vi "Autonomous Independent.vi"() -> ()   [LabVIEW 2014]
doc: "This VI is called when autonomous begins, and will automatically be terminated when autonomous ends. You can carry out timed or sensor driven robot movement independently without needing to return to the caller."
uses:
  <vilib>/Rock Robotics/WPI/Joystick/WPI_JoystickGetSetRefNum.vi
  <vilib>/Rock Robotics/WPI/RobotDrive/WPI_RobotDriveGetSetRefNum.vi
  Robot Global Data.vi
  <vilib>/Rock Robotics/WPI/RobotDrive/WPI_RobotDriveArcadeDrive_Standard(NoSaturation).vi
  <vilib>/Rock Robotics/Network Tables/SD Write Boolean.vi
panel:
  out "Auto 6":bool=TRUE
  out "Auto 5":bool=TRUE
  in  "Array of robot movements 6":T1(array[cluster])=[{"X Joystick Value"=0.7, "Y Joystick Value"=0.0, "Delay (sec)"=2.0, "Movement Name"="90 turn", "Joystick Button 1"=FALSE, "Joystick Button 2"=FALSE, "Joystick Button 3"=FALSE, "Joystick Button 4"=FALSE, "Joystick Button 5"=FALSE, "Joystick Button 6"=FALSE, "Joystick Button 7"=FALSE, "Joystick Button 8"=FALSE, "Joystick Button 9"=FALSE, "Joystick Button 10"=FALSE, "Joystick Button 11"=FALSE, "Joystick Button 12"=FALSE}, {"X Joystick Value"=0.0, "Y Joystick Value"=0.0, "Delay (sec)"=0.0, "Movement Name"="Stop", "Joystick Button 1"=FALSE, "Joystick Button 2"=FALSE, "Joystick Button 3"=FALSE, "Joystick Button 4"=FALSE, "Joystick Button 5"=FALSE, "Joystick Button 6"=FALSE, "Joystick Button 7"=FALSE, "Joystick Button 8"=FALSE, "Joystick Button 9"=FALSE, "Joystick Button 10"=FALSE, "Joystick Button 11"=FALSE, "Joystick Button 12"=FALSE}] {"Y Joystick Value" scale=1.0..-1.0; "X Joystick Value" scale=-1.0..1.0}
  in  "Array of robot movements 5":T1(array[cluster])=[{"X Joystick Value"=0.17, "Y Joystick Value"=-0.45, "Delay (sec)"=1.2, "Movement Name"="Drive 600mm", "Joystick Button 1"=FALSE, "Joystick Button 2"=FALSE, "Joystick Button 3"=FALSE, "Joystick Button 4"=FALSE, "Joystick Button 5"=FALSE, "Joystick Button 6"=FALSE, "Joystick Button 7"=FALSE, "Joystick Button 8"=FALSE, "Joystick Button 9"=FALSE, "Joystick Button 10"=FALSE, "Joystick Button 11"=FALSE, "Joystick Button 12"=FALSE}, {"X Joystick Value"=0.0, "Y Joystick Value"=0.0, "Delay (sec)"=0.0, "Movement Name"="Stop", "Joystick Button 1"=FALSE, "Joystick Button 2"=FALSE, "Joystick Button 3"=FALSE, "Joystick Button 4"=FALSE, "Joystick Button 5"=FALSE, "Joystick Button 6"=FALSE, "Joystick Button 7"=FALSE, "Joystick Button 8"=FALSE, "Joystick Button 9"=FALSE, "Joystick Button 10"=FALSE, "Joystick Button 11"=FALSE, "Joystick Button 12"=FALSE}] {"Y Joystick Value" scale=1.0..-1.0; "X Joystick Value" scale=-1.0..1.0}
  out "Auto 4":bool=TRUE
  out "Auto 3":bool=TRUE
  out "Auto 2":bool=TRUE
  out "Auto 1":bool=TRUE
  in  "Array of robot movements 4":T1(array[cluster])=[{"X Joystick Value"=0.33, "Y Joystick Value"=-0.75, "Delay (sec)"=5.0, "Movement Name"="Drive to Auto", "Joystick Button 1"=FALSE, "Joystick Button 2"=FALSE, "Joystick Button 3"=FALSE, "Joystick Button 4"=FALSE, "Joystick Button 5"=FALSE, "Joystick Button 6"=FALSE, "Joystick Button 7"=FALSE, "Joystick Button 8"=FALSE, "Joystick Button 9"=FALSE, "Joystick Button 10"=FALSE, "Joystick Button 11"=FALSE, "Joystick Button 12"=FALSE}, {"X Joystick Value"=0.0, "Y Joystick Value"=0.0, "Delay (sec)"=0.0, "Movement Name"="Stop", "Joystick Button 1"=FALSE, "Joystick Button 2"=FALSE, "Joystick Button 3"=FALSE, "Joystick Button 4"=FALSE, "Joystick Button 5"=FALSE, "Joystick Button 6"=FALSE, "Joystick Button 7"=FALSE, "Joystick Button 8"=FALSE, "Joystick Button 9"=FALSE, "Joystick Button 10"=FALSE, "Joystick Button 11"=FALSE, "Joystick Button 12"=FALSE}] {"Y Joystick Value" scale=1.0..-1.0; "X Joystick Value" scale=-1.0..1.0}
  in  "Array of robot movements 3":T1(array[cluster])=[{"X Joystick Value"=0.7, "Y Joystick Value"=0.0, "Delay (sec)"=1.4, "Movement Name"="Turn 90' right", "Joystick Button 1"=FALSE, "Joystick Button 2"=FALSE, "Joystick Button 3"=FALSE, "Joystick Button 4"=FALSE, "Joystick Button 5"=FALSE, "Joystick Button 6"=FALSE, "Joystick Button 7"=FALSE, "Joystick Button 8"=FALSE, "Joystick Button 9"=FALSE, "Joystick Button 10"=FALSE, "Joystick Button 11"=FALSE, "Joystick Button 12"=FALSE}, {"X Joystick Value"=0.33, "Y Joystick Value"=-0.75, "Delay (sec)"=3.0, "Movement Name"="Drive to Auto", "Joystick Button 1"=FALSE, "Joystick Button 2"=FALSE, "Joystick Button 3"=FALSE, "Joystick Button 4"=FALSE, "Joystick Button 5"=FALSE, "Joystick Button 6"=FALSE, "Joystick Button 7"=FALSE, "Joystick Button 8"=FALSE, "Joystick Button 9"=FALSE, "Joystick Button 10"=FALSE, "Joystick Button 11"=FALSE, "Joystick Button 12"=FALSE}, {"X Joystick Value"=0.0, "Y Joystick Value"=0.0, "Delay (sec)"=0.0, "Movement Name"="Stop", "Joystick Button 1"=FALSE, "Joystick Button 2"=FALSE, "Joystick Button 3"=FALSE, "Joystick Button 4"=FALSE, "Joystick Button 5"=FALSE, "Joystick Button 6"=FALSE, "Joystick Button 7"=FALSE, "Joystick Button 8"=FALSE, "Joystick Button 9"=FALSE, "Joystick Button 10"=FALSE, "Joystick Button 11"=FALSE, "Joystick Button 12"=FALSE}] {"Y Joystick Value" scale=1.0..-1.0; "X Joystick Value" scale=-1.0..1.0}
  in  "Array of robot movements 2":T1(array[cluster])=[{"X Joystick Value"=0.0, "Y Joystick Value"=0.0, "Delay (sec)"=0.5, "Movement Name"="Lift arm 4 bin", "Joystick Button 1"=FALSE, "Joystick Button 2"=FALSE, "Joystick Button 3"=FALSE, "Joystick Button 4"=FALSE, "Joystick Button 5"=FALSE, "Joystick Button 6"=FALSE, "Joystick Button 7"=FALSE, "Joystick Button 8"=TRUE, "Joystick Button 9"=FALSE, "Joystick Button 10"=FALSE, "Joystick Button 11"=FALSE, "Joystick Button 12"=FALSE}, {"X Joystick Value"=0.0, "Y Joystick Value"=0.0, "Delay (sec)"=4.55, "Movement Name"="Wait for arm", "Joystick Button 1"=FALSE, "Joystick Button 2"=FALSE, "Joystick Button 3"=FALSE, "Joystick Button 4"=FALSE, "Joystick Button 5"=FALSE, "Joystick Button 6"=FALSE, "Joystick Button 7"=FALSE, "Joystick Button 8"=FALSE, "Joystick Button 9"=FALSE, "Joystick Button 10"=FALSE, "Joystick Button 11"=FALSE, "Joystick Button 12"=FALSE}, {"X Joystick Value"=0.33, "Y Joystick Value"=-0.75, "Delay (sec)"=5.0, "Movement Name"="Drive to Auto", "Joystick Button 1"=FALSE, "Joystick Button 2"=FALSE, "Joystick Button 3"=FALSE, "Joystick Button 4"=FALSE, "Joystick Button 5"=FALSE, "Joystick Button 6"=FALSE, "Joystick Button 7"=FALSE, "Joystick Button 8"=FALSE, "Joystick Button 9"=FALSE, "Joystick Button 10"=FALSE, "Joystick Button 11"=FALSE, "Joystick Button 12"=FALSE}, {"X Joystick Value"=0.0, "Y Joystick Value"=0.0, "Delay (sec)"=0.0, "Movement Name"="Stop", "Joystick Button 1"=FALSE, "Joystick Button 2"=FALSE, "Joystick Button 3"=FALSE, "Joystick Button 4"=FALSE, "Joystick Button 5"=FALSE, "Joystick Button 6"=FALSE, "Joystick Button 7"=FALSE, "Joystick Button 8"=FALSE, "Joystick Button 9"=FALSE, "Joystick Button 10"=FALSE, "Joystick Button 11"=FALSE, "Joystick Button 12"=FALSE}] {"Y Joystick Value" scale=1.0..-1.0; "X Joystick Value" scale=-1.0..1.0}
  in  "Array of robot movements 1":T1(array[cluster])=[{"X Joystick Value"=0.0, "Y Joystick Value"=0.0, "Delay (sec)"=0.5, "Movement Name"="lift arm 4 bin", "Joystick Button 1"=FALSE, "Joystick Button 2"=FALSE, "Joystick Button 3"=FALSE, "Joystick Button 4"=FALSE, "Joystick Button 5"=FALSE, "Joystick Button 6"=FALSE, "Joystick Button 7"=FALSE, "Joystick Button 8"=TRUE, "Joystick Button 9"=FALSE, "Joystick Button 10"=FALSE, "Joystick Button 11"=FALSE, "Joystick Button 12"=FALSE}, {"X Joystick Value"=0.0, "Y Joystick Value"=0.0, "Delay (sec)"=4.55, "Movement Name"="Wait for arm", "Joystick Button 1"=FALSE, "Joystick Button 2"=FALSE, "Joystick Button 3"=FALSE, "Joystick Button 4"=FALSE, "Joystick Button 5"=FALSE, "Joystick Button 6"=FALSE, "Joystick Button 7"=FALSE, "Joystick Button 8"=FALSE, "Joystick Button 9"=FALSE, "Joystick Button 10"=FALSE, "Joystick Button 11"=FALSE, "Joystick Button 12"=FALSE}, {"X Joystick Value"=0.7, "Y Joystick Value"=0.0, "Delay (sec)"=1.4, "Movement Name"="Turn 90 right", "Joystick Button 1"=FALSE, "Joystick Button 2"=FALSE, "Joystick Button 3"=FALSE, "Joystick Button 4"=FALSE, "Joystick Button 5"=FALSE, "Joystick Button 6"=FALSE, "Joystick Button 7"=FALSE, "Joystick Button 8"=FALSE, "Joystick Button 9"=FALSE, "Joystick Button 10"=FALSE, "Joystick Button 11"=FALSE, "Joystick Button 12"=FALSE}, {"X Joystick Value"=0.33, "Y Joystick Value"=-0.75, "Delay (sec)"=3.0, "Movement Name"="Drive to Auto", "Joystick Button 1"=FALSE, "Joystick Button 2"=FALSE, "Joystick Button 3"=FALSE, "Joystick Button 4"=FALSE, "Joystick Button 5"=FALSE, "Joystick Button 6"=FALSE, "Joystick Button 7"=FALSE, "Joystick Button 8"=FALSE, "Joystick Button 9"=FALSE, "Joystick Button 10"=FALSE, "Joystick Button 11"=FALSE, "Joystick Button 12"=FALSE}, {"X Joystick Value"=0.0, "Y Joystick Value"=0.0, "Delay (sec)"=0.0, "Movement Name"="Stop", "Joystick Button 1"=FALSE, "Joystick Button 2"=FALSE, "Joystick Button 3"=FALSE, "Joystick Button 4"=FALSE, "Joystick Button 5"=FALSE, "Joystick Button 6"=FALSE, "Joystick Button 7"=FALSE, "Joystick Button 8"=FALSE, "Joystick Button 9"=FALSE, "Joystick Button 10"=FALSE, "Joystick Button 11"=FALSE, "Joystick Button 12"=FALSE}] {"Y Joystick Value" scale=1.0..-1.0; "X Joystick Value" scale=-1.0..1.0}
  # "######################################################\n    #                                                      #\n    #   SAFETY NOTICE: MAKE SURE THAT EACH ARRAY ON THIS   #\n    #   FRONT PANEL IS DISPLAYING A \"GREYED OUT\" (DEFAULT) #\n    #   ELEMENT ON THE RIGHT                               #\n    #                                                      #\n     ######################################################\n\nNOTE#1: any changes made here are not permanent until you have selected the modified array, right-click and select \"Data Operations\" > \"Make Current Value Default\"\n\nNOTE#2: to add an extra \"element\" to one of the arrays simply select the array and drag the right side further to the right, a new element will be added to the end of the array. Alternatively, select an existing element then right click and select \"Data Operations\" > \"Insert Element Before\".\n\nNOTE#3: to remove an element you must explicitly delete the element, DO NOT be tempted to just grab the end of the array and drag it to the left as all that does is limit what is visible on screen. To delete an element select it then right-click and select \"Data Operations\" > \"Delete Element\"."
  # "AUTO 1:\n1 bin\n1 tote"
  # "Start around left bin\nwith arm down"
  # "AUTO 2:\n1 bin\n2 totes"
  # "starts around middle bin\nwith arm down"
  # "AUTO 3:\nReady 1 tote"
  # "Starts around left tote\nwith arm down"
  # "Be sure to right-click and choose Data Operations>>Make Current Value default if you want to save the array values with the VI"
  # "AUTO 4:\nAuto Zone"
  # "Start backed up to left tote\nArm doesn't matter"
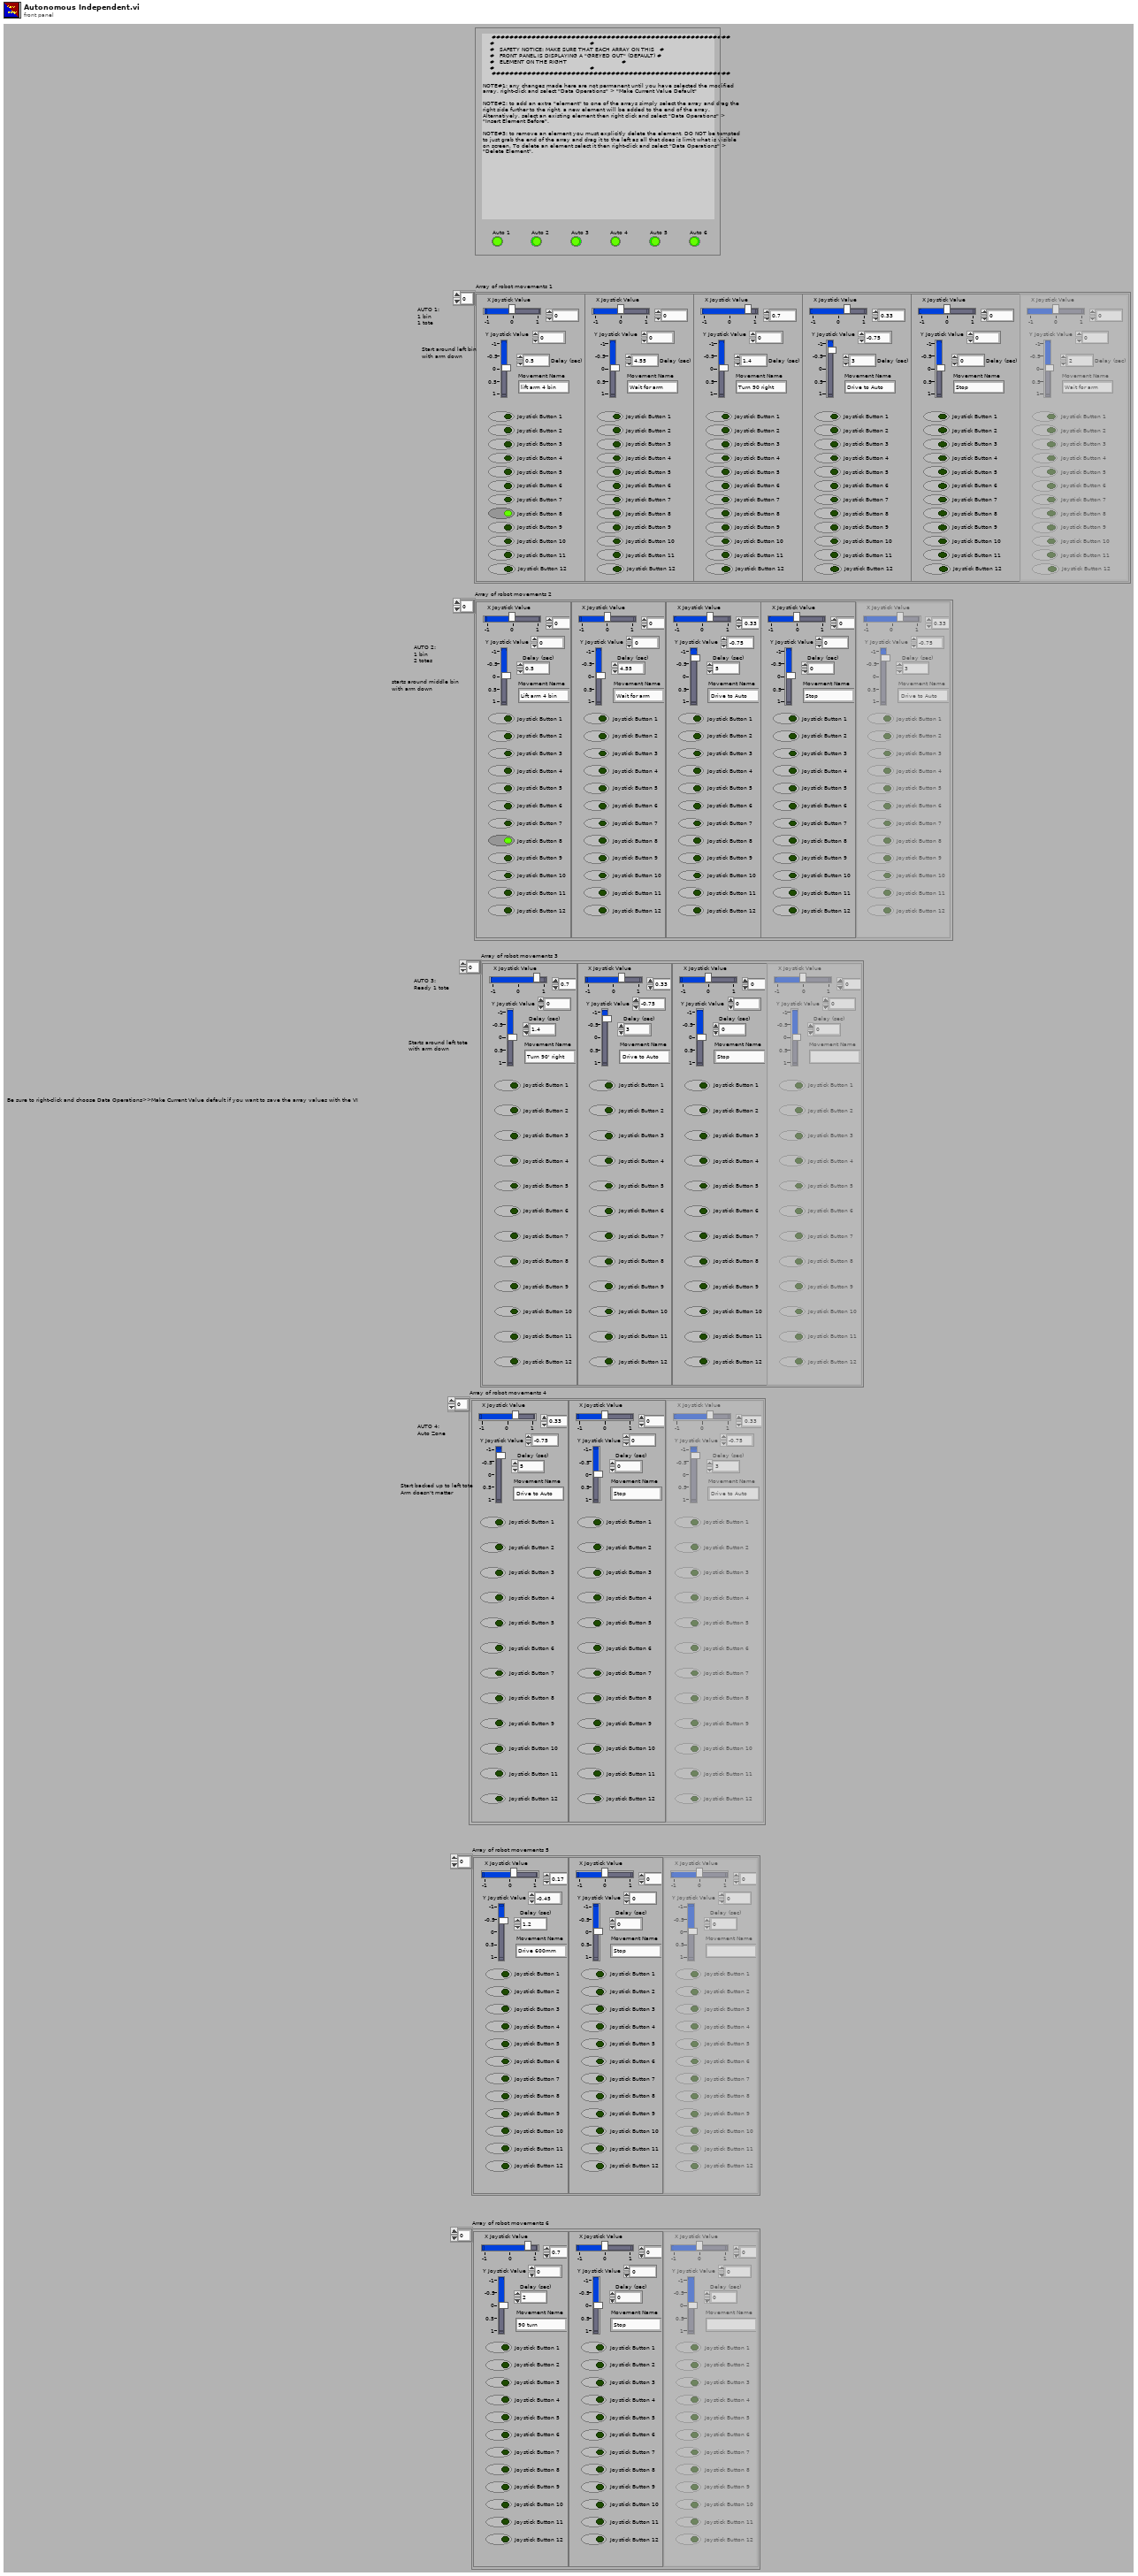
[diagram p1: front panel]
types:
  T1 = cluster{"X Joystick Value":dbl, "Y Joystick Value":dbl, "Delay (sec)":dbl, "Movement Name":string, "Joystick Button 1":bool, "Joystick Button 2":bool, "Joystick Button 3":bool, "Joystick Button 4":bool, "Joystick Button 5":bool, "Joystick Button 6":bool, "Joystick Button 7":bool, "Joystick Button 8":bool, "Joystick Button 9":bool, "Joystick Button 10":bool, "Joystick Button 11":bool, "Joystick Button 12":bool}[]
  T2 = typedef "WPI_JoystickDevRef.ctl" = cluster{"Device":T3}
  T3 = typedef "WPI_JoystickDeviceEnum.ctl" = enum16{"USB 0", "USB 1", "USB 2", "USB 3", "USB 4", "USB 5"}
  T4 = typedef "WPI_DigitalInputDevRef.ctl" = cluster{"DevStatus":errorcluster, "DIO Channel":T5, "Controller":T6}
  T5 = typedef "FPGA_DIOChannel.ctl" = enum8{"DIO 0", "DIO 1", "DIO 2", "DIO 3", "DIO 4", "DIO 5", "DIO 6", "DIO 7", "DIO 8", "DIO 9", "DIO MXP 0", "DIO MXP 1", "DIO MXP 2", "DIO MXP 3", "DIO MXP 4", "DIO MXP 5", "DIO MXP 6", "DIO MXP 7", "DIO MXP 8", "DIO MXP 9", "DIO MXP 10", "DIO MXP 11", "DIO MXP 12", "DIO MXP 13", "DIO MXP 14", "DIO MXP 15", "Invalid"}
  T6 = typedef "FPGA_TypedefDigitalModule.ctl" = enum16{"Controller 1"}
  T7 = typedef "WPI_RobotDriveDevRef.ctl" = cluster{"DevStatus":errorcluster, "Motors[]":T8[], "Square Inputs":bool, "Max Output":dbl}
  T8 = typedef "WPI_MotorControlDeviceRef.ctl" = cluster{"DeviceStatus":errorcluster, "Type":T9, "PWM":cluster{"Controller":T6, "PWM Channel":T10, "DeadBand":T11}, "CAN":cluster{"Device Number":u8, "Control Mode":T12, "Semaphore":T13, "Max Vout":dbl, "TalonSRX Control Mode":T14}, "Invert":bool, "TransformRef":T15, "InvTransformRef":T15}
  T9 = typedef "WPI_MotorControlType.ctl" = enum16{"PWM", "CAN", "CANTalonSRX"}
  T10 = typedef "FPGA_DIOPWMChannel.ctl" = enum8{"PWM 0", "PWM 1", "PWM 2", "PWM 3", "PWM 4", "PWM 5", "PWM 6", "PWM 7", "PWM 8", "PWM 9", "PWM MXP 0", "PWM MXP 1", "PWM MXP 2", "PWM MXP 3", "PWM MXP 4", "PWM MXP 5", "PWM MXP 6", "PWM MXP 7", "PWM MXP 8", "PWM MXP 9", "Invalid"}
  T11 = typedef "WPI_PWMDeadband.ctl" = cluster{"Name":string, "maxPositivePwm":i32, "minPositivePwm":i32, "centerPwm":i32, "maxNegativePwm":i32, "minNegativePwm":i32, "angularRange":u16}
  T12 = typedef "WPI_CANJaguar_ControlMode.ctl" = enum8{"Percent VBus", "Current", "Speed", "Position", "Voltage"}
  T13 = typedef "Semaphore RefNum" = refnum<k1>
  T14 = typedef "WPI_CANTalonSRX_APIControlMode.ctl" = enum8{"Percent VBus", "Speed", "Position", "Slave", "Unchanged / Invalid"}
  T15 = typedef "WPI_PWMTransform_ConPane.ctl" = refnum<vi>
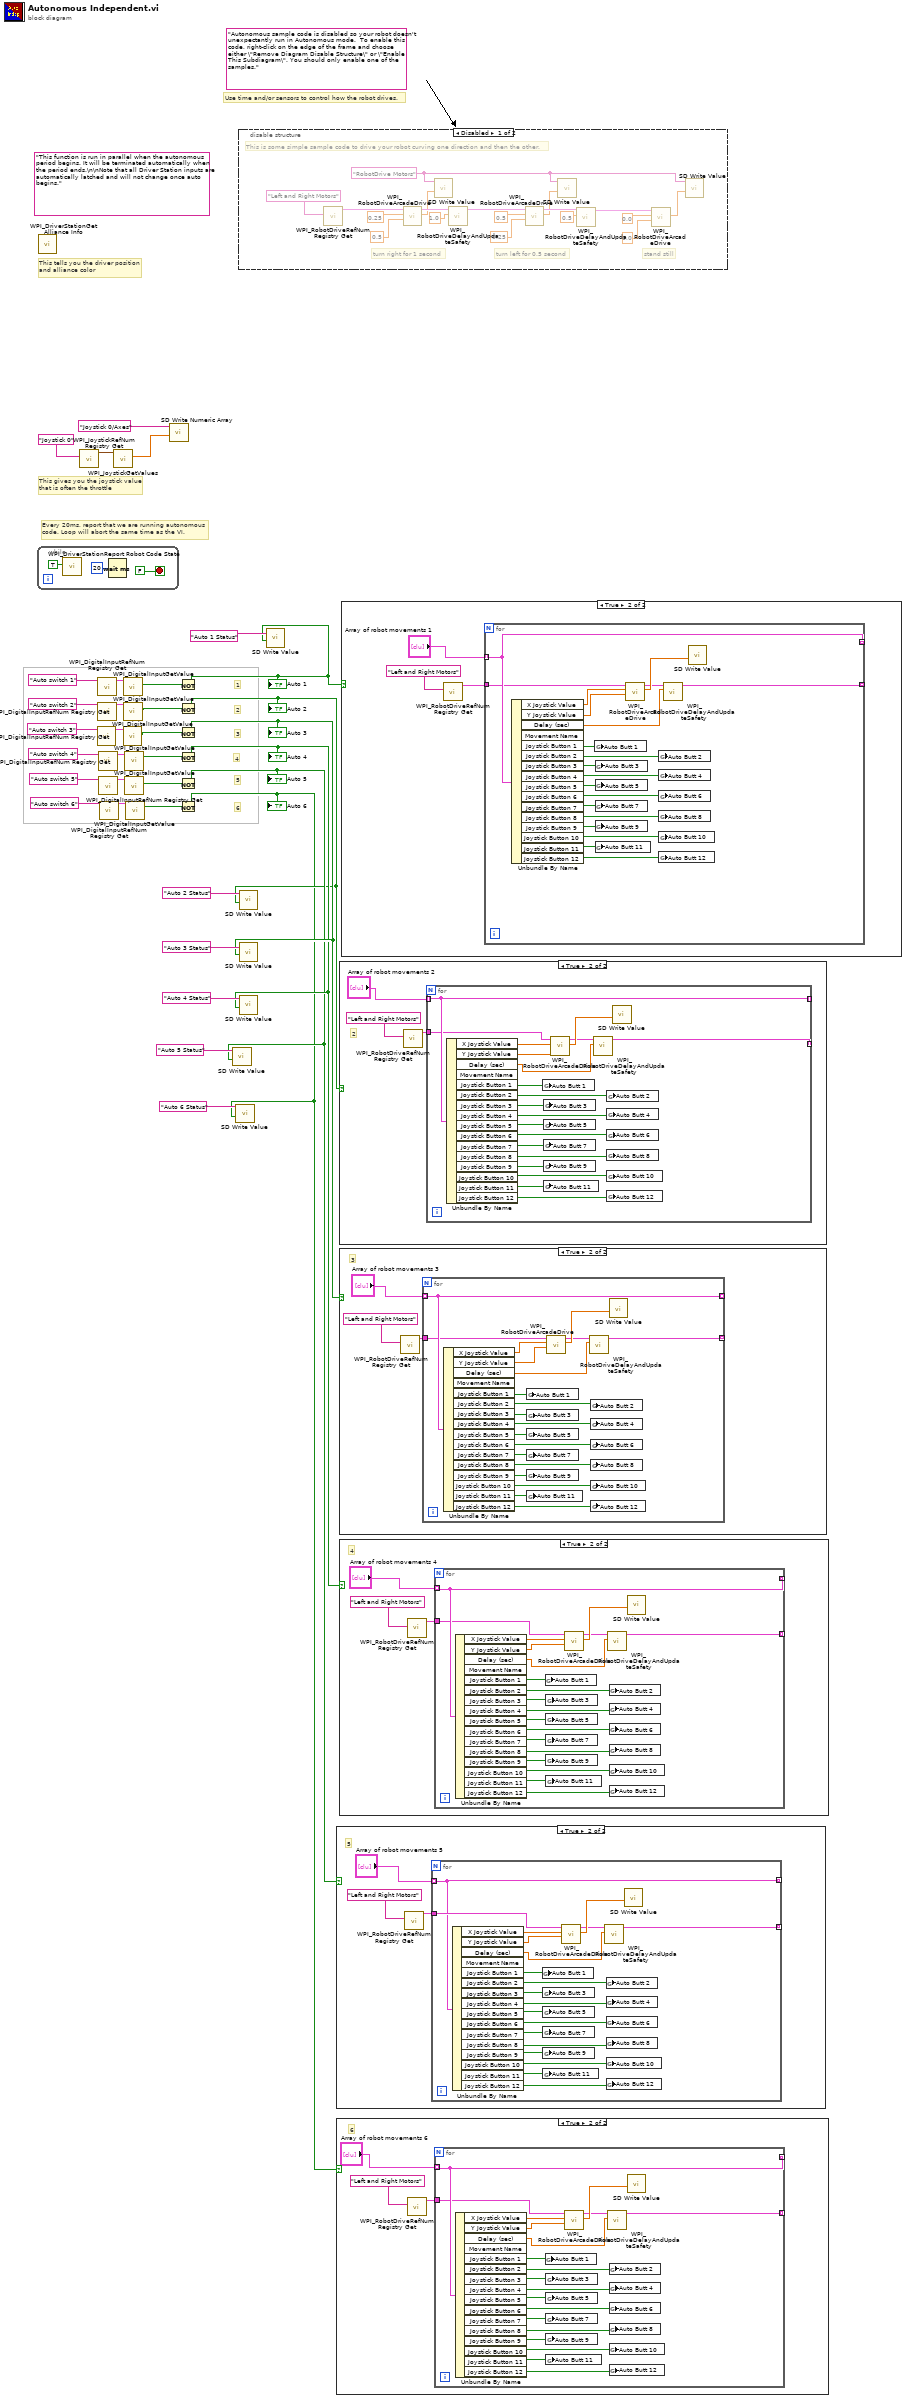
[diagram p0: block diagram]
diagram:
  (unwired) "Autonomous sample code is disabled so your robot doesn't unexpectantly run in Autonomous mode.  To enable this code, right-click on the edge of the frame and choose either \"Remove Diagram Disable Structure\" or \"Enable This Subdiagram\". You should only enable one of the samples."
  (unwired) "This function is run in parallel when the autonomous period begins. It will be terminated automatically when the period ends.\n\nNote that all Driver Station inputs are automatically latched and will not change once auto begins."
  # "6"
  # "5"
  # "4"
  # "3"
  # "2"
  # "1"
  # "Every 20ms, report that we are running autonomous\ncode. Loop will abort the same time as the VI."
  # "This gives you the joystick value\nthat is often the throttle"
  # "Use time and/or sensors to control how the robot drives."
  # "This tells you the driver position\nand alliance color"
  n1 = while {
    stop <- FALSE stop-if-true
    n2 = call <vilib>:"WPI_DriverStationReport Robot Code State.vi"("Autonomous"=TRUE) -> ()  [unwired: 10 in, 1 out]
    n3 = Wait (ms)(milliseconds to wait=u32 20) -> ()  [unwired: 1 out]
  }
  n4 = call <vilib>:"WPI_DriverStationGet Alliance Info.vi"() -> ()  [unwired: 12 out]
  n5 = call <vilib>:"WPI_JoystickRefNum Registry Get.vi"("refnum name"="Joystick 0") -> ("JoystickDevRef"=w33:T2)  [unwired: 1 in, 9 out]
  n6 = call <vilib>:"WPI_DigitalInputRefNum Registry Get.vi"("refnum name"="Auto switch 3") -> ("DigitalInputDevRef"=w15:T4)  [unwired: 9 in, 1 out]
  n7 = call <vilib>:"WPI_DigitalInputRefNum Registry Get.vi"("refnum name"="Auto switch 1") -> ("DigitalInputDevRef"=w27:T4)  [unwired: 9 in, 1 out]
  n8 = call <vilib>:"WPI_DigitalInputRefNum Registry Get.vi"("refnum name"="Auto switch 2") -> ("DigitalInputDevRef"=w28:T4)  [unwired: 9 in, 1 out]
  n9 = call <vilib>:"WPI_DigitalInputRefNum Registry Get.vi"("refnum name"="Auto switch 4") -> ("DigitalInputDevRef"=w16:T4)  [unwired: 9 in, 1 out]
  n10 = call <vilib>:"WPI_DigitalInputRefNum Registry Get.vi"("refnum name"="Auto switch 5") -> ("DigitalInputDevRef"=w14:T4)  [unwired: 9 in, 1 out]
  n11 = call <vilib>:"WPI_DigitalInputRefNum Registry Get.vi"("refnum name"="Auto switch 6") -> ("DigitalInputDevRef"=w13:T4)  [unwired: 9 in, 1 out]
  n12 = call <vilib>:"WPI_JoystickGetValues.vi"("JoystickDevRef"=w33) -> ("Axes"=w31:dbl[])  [unwired: 6 in, 4 out]
  n13 = call <vilib>:"WPI_DigitalInputGetValue.vi"("DigitalInputDevRef"=w15) -> ("Value"=w10:bool)  [unwired: 8 in, 2 out]
  n14 = call <vilib>:"WPI_DigitalInputGetValue.vi"("DigitalInputDevRef"=w27) -> ("Value"=w12:bool)  [unwired: 8 in, 2 out]
  n15 = call <vilib>:"WPI_DigitalInputGetValue.vi"("DigitalInputDevRef"=w28) -> ("Value"=w11:bool)  [unwired: 8 in, 2 out]
  n16 = call <vilib>:"WPI_DigitalInputGetValue.vi"("DigitalInputDevRef"=w16) -> ("Value"=w8:bool)  [unwired: 8 in, 2 out]
  n17 = call <vilib>:"WPI_DigitalInputGetValue.vi"("DigitalInputDevRef"=w14) -> ("Value"=w6:bool)  [unwired: 8 in, 2 out]
  n18 = call <vilib>:"WPI_DigitalInputGetValue.vi"("DigitalInputDevRef"=w13) -> ("Value"=w4:bool)  [unwired: 8 in, 2 out]
  n19 = call <vilib>:"SD Write Numeric Array.vi"("Numeric Array"=w31, "Name"="Joystick 0/Axes") -> ()  [unwired: 8 in, 2 out]
  n20 = Not(x=w12) -> (.not. x?=w3:bool)
  "Auto 1" <- w3
  n21 = Not(x=w11) -> (.not. x?=w2:bool)
  "Auto 2" <- w2
  n22 = Not(x=w10) -> (.not. x?=w9:bool)
  "Auto 3" <- w9
  n23 = Not(x=w8) -> (.not. x?=w7:bool)
  "Auto 4" <- w7
  n24 = Not(x=w6) -> (.not. x?=w5:bool)
  "Auto 5" <- w5
  n25 = Not(x=w4) -> (.not. x?=w1:bool)
  "Auto 6" <- w1
  n26 = call-poly <vilib>:"SD Write Value.vi"("Boolean"=w5, "Name"="Auto 5 Status") -> ()  [unwired: 8 in, 2 out]
  n27 = call-poly <vilib>:"SD Write Value.vi"("Boolean"=w1, "Name"="Auto 6 Status") -> ()  [unwired: 8 in, 2 out]
  n28 = disable-structure shown="Disabled" {
    frame Disabled {
      w41 = "RobotDrive Motors" ("Name")
      # "This is some simple sample code to drive your robot curving one direction and then the other."
      # "stand still"
      # "turn left for 0.5 second"
      # "turn right for 1 second"
      n29 = call <vilib>:"WPI_RobotDriveRefNum Registry Get.vi"("refnum name"="Left and Right Motors") -> ("RobotDriveDevRef"=w42:T7)  [unwired: 1 in, 9 out]
      n30 = call-poly <vilib>:"WPI_RobotDriveArcadeDrive.vi"("Y axis value"=0.5 ("X axis value"), "X axis value"=0.25, "RobotDriveDevRef"=w42) -> ("Motor Values"=w40:dbl[], "RobotDriveDevRef"=w49:T7)  [unwired: 1 in, 6 out]
      n31 = call-poly <vilib>:"SD Write Value.vi"("Numeric Array"=w40, "Name"=w41) -> ()  [unwired: 8 in, 2 out]
      n32 = call <vilib>:"WPI_RobotDriveDelayAndUpdateSafety.vi"("Delay (s)"=1.0, "RobotDriveDevRef"=w49) -> ("RobotDriveDevRef 2"=w48:T7)  [unwired: 8 in, 1 out]
      n33 = call-poly <vilib>:"WPI_RobotDriveArcadeDrive.vi"("Y axis value"=0.25 ("X axis value"), "X axis value"=0.5, "RobotDriveDevRef"=w48) -> ("Motor Values"=w39:dbl[], "RobotDriveDevRef"=w47:T7)  [unwired: 1 in, 6 out]
      n34 = call-poly <vilib>:"SD Write Value.vi"("Numeric Array"=w39, "Name"=w41) -> ()  [unwired: 8 in, 2 out]
      n35 = call <vilib>:"WPI_RobotDriveDelayAndUpdateSafety.vi"("Delay (s)"=0.5, "RobotDriveDevRef"=w47) -> ("RobotDriveDevRef 2"=w46:T7)  [unwired: 8 in, 1 out]
      n36 = call-poly <vilib>:"WPI_RobotDriveArcadeDrive.vi"("Y axis value"=0.0 ("X axis value"), "X axis value"=0.0, "RobotDriveDevRef"=w46) -> ("Motor Values"=w38:dbl[])  [unwired: 1 in, 7 out]
      n37 = call-poly <vilib>:"SD Write Value.vi"("Numeric Array"=w38, "Name"=w41) -> ()  [unwired: 8 in, 2 out]
    }
    frame Enabled {
    }
  }
  n38 = call-poly <vilib>:"SD Write Value.vi"("Boolean"=w2, "Name"="Auto 2 Status") -> ()  [unwired: 8 in, 2 out]
  n39 = call-poly <vilib>:"SD Write Value.vi"("Boolean"=w9, "Name"="Auto 3 Status") -> ()  [unwired: 8 in, 2 out]
  n40 = call-poly <vilib>:"SD Write Value.vi"("Boolean"=w7, "Name"="Auto 4 Status") -> ()  [unwired: 8 in, 2 out]
  n41 = call-poly <vilib>:"SD Write Value.vi"("Boolean"=w3, "Name"="Auto 1 Status") -> ()  [unwired: 8 in, 2 out]
  n42 = case shown="True" w5 {
    frame False {
    }
    frame True {
      # "5"
      n43 = call <vilib>:"WPI_RobotDriveRefNum Registry Get.vi"("refnum name"="Left and Right Motors") -> ("RobotDriveDevRef"=w57:T7)  [unwired: 1 in, 9 out]
      n44 = for {
        tunnel: "Array of robot movements 5" -> [w59] mode=indexing
        tunnel: [w59] -> _ mode=indexing
        tunnel: w57 -> [w76]
        tunnel: [w73] -> _ mode=indexing
        n45 = Unbundle By Name(w59) -> ("X Joystick Value"=w75:dbl, "Y Joystick Value"=w74:dbl, "Delay (sec)"=w72:dbl, "Joystick Button 1"=w71:bool, "Joystick Button 2"=w65:bool, "Joystick Button 3"=w70:bool, "Joystick Button 4"=w64:bool, "Joystick Button 5"=w69:bool, "Joystick Button 6"=w63:bool, "Joystick Button 7"=w68:bool, "Joystick Button 8"=w62:bool, "Joystick Button 9"=w67:bool, "Joystick Button 10"=w61:bool, "Joystick Button 11"=w66:bool, "Joystick Button 12"=w60:bool)  [unwired: 1 out]
        n46 = global write "Robot Global Data.vi" "Auto Butt 1"(w71) -> ()
        n47 = global write "Robot Global Data.vi" "Auto Butt 3"(w70) -> ()
        n48 = global write "Robot Global Data.vi" "Auto Butt 5"(w69) -> ()
        n49 = global write "Robot Global Data.vi" "Auto Butt 7"(w68) -> ()
        n50 = global write "Robot Global Data.vi" "Auto Butt 9"(w67) -> ()
        n51 = global write "Robot Global Data.vi" "Auto Butt 11"(w66) -> ()
        n52 = call-poly <vilib>:"WPI_RobotDriveArcadeDrive.vi"("Y axis value"=w74, "X axis value"=w75, "RobotDriveDevRef"=w76) -> ("Motor Values"=w78:dbl[], "RobotDriveDevRef"=w77:T7)  [unwired: 1 in, 6 out]
        n53 = call <vilib>:"WPI_RobotDriveDelayAndUpdateSafety.vi"("Delay (s)"=w72, "RobotDriveDevRef"=w77) -> ("RobotDriveDevRef 2"=w73:T7)  [unwired: 8 in, 1 out]
        n54 = global write "Robot Global Data.vi" "Auto Butt 2"(w65) -> ()
        n55 = global write "Robot Global Data.vi" "Auto Butt 4"(w64) -> ()
        n56 = global write "Robot Global Data.vi" "Auto Butt 6"(w63) -> ()
        n57 = global write "Robot Global Data.vi" "Auto Butt 8"(w62) -> ()
        n58 = global write "Robot Global Data.vi" "Auto Butt 10"(w61) -> ()
        n59 = global write "Robot Global Data.vi" "Auto Butt 12"(w60) -> ()
        n60 = call-poly <vilib>:"SD Write Value.vi"("Numeric Array"=w78) -> ()  [unwired: 9 in, 2 out]
      }
    }
  }
  n61 = case shown="True" w1 {
    frame False {
    }
    frame True {
      # "6"
      n62 = call <vilib>:"WPI_RobotDriveRefNum Registry Get.vi"("refnum name"="Left and Right Motors") -> ("RobotDriveDevRef"=w80:T7)  [unwired: 1 in, 9 out]
      n63 = for {
        tunnel: "Array of robot movements 6" -> [w101] mode=indexing
        tunnel: [w101] -> _ mode=indexing
        tunnel: w80 -> [w98]
        tunnel: [w95] -> _ mode=indexing
        n64 = Unbundle By Name(w101) -> ("X Joystick Value"=w97:dbl, "Y Joystick Value"=w96:dbl, "Delay (sec)"=w94:dbl, "Joystick Button 1"=w93:bool, "Joystick Button 2"=w87:bool, "Joystick Button 3"=w92:bool, "Joystick Button 4"=w86:bool, "Joystick Button 5"=w91:bool, "Joystick Button 6"=w85:bool, "Joystick Button 7"=w90:bool, "Joystick Button 8"=w84:bool, "Joystick Button 9"=w89:bool, "Joystick Button 10"=w83:bool, "Joystick Button 11"=w88:bool, "Joystick Button 12"=w82:bool)  [unwired: 1 out]
        n65 = global write "Robot Global Data.vi" "Auto Butt 1"(w93) -> ()
        n66 = global write "Robot Global Data.vi" "Auto Butt 3"(w92) -> ()
        n67 = global write "Robot Global Data.vi" "Auto Butt 5"(w91) -> ()
        n68 = global write "Robot Global Data.vi" "Auto Butt 7"(w90) -> ()
        n69 = global write "Robot Global Data.vi" "Auto Butt 9"(w89) -> ()
        n70 = global write "Robot Global Data.vi" "Auto Butt 11"(w88) -> ()
        n71 = call-poly <vilib>:"WPI_RobotDriveArcadeDrive.vi"("Y axis value"=w96, "X axis value"=w97, "RobotDriveDevRef"=w98) -> ("Motor Values"=w100:dbl[], "RobotDriveDevRef"=w99:T7)  [unwired: 1 in, 6 out]
        n72 = call <vilib>:"WPI_RobotDriveDelayAndUpdateSafety.vi"("Delay (s)"=w94, "RobotDriveDevRef"=w99) -> ("RobotDriveDevRef 2"=w95:T7)  [unwired: 8 in, 1 out]
        n73 = global write "Robot Global Data.vi" "Auto Butt 2"(w87) -> ()
        n74 = global write "Robot Global Data.vi" "Auto Butt 4"(w86) -> ()
        n75 = global write "Robot Global Data.vi" "Auto Butt 6"(w85) -> ()
        n76 = global write "Robot Global Data.vi" "Auto Butt 8"(w84) -> ()
        n77 = global write "Robot Global Data.vi" "Auto Butt 10"(w83) -> ()
        n78 = global write "Robot Global Data.vi" "Auto Butt 12"(w82) -> ()
        n79 = call-poly <vilib>:"SD Write Value.vi"("Numeric Array"=w100) -> ()  [unwired: 9 in, 2 out]
      }
    }
  }
  n80 = case shown="True" w2 {
    frame False {
    }
    frame True {
      # "2"
      n81 = call <vilib>:"WPI_RobotDriveRefNum Registry Get.vi"("refnum name"="Left and Right Motors") -> ("RobotDriveDevRef"=w102:T7)  [unwired: 1 in, 9 out]
      n82 = for {
        tunnel: [w124] -> _ mode=indexing
        tunnel: "Array of robot movements 2" -> [w124] mode=indexing
        tunnel: w102 -> [w119]
        tunnel: [w118] -> _ mode=indexing
        n83 = Unbundle By Name(w124) -> ("X Joystick Value"=w121:dbl, "Y Joystick Value"=w120:dbl, "Delay (sec)"=w117:dbl, "Joystick Button 1"=w116:bool, "Joystick Button 2"=w105:bool, "Joystick Button 3"=w115:bool, "Joystick Button 4"=w106:bool, "Joystick Button 5"=w114:bool, "Joystick Button 6"=w107:bool, "Joystick Button 7"=w113:bool, "Joystick Button 8"=w108:bool, "Joystick Button 9"=w112:bool, "Joystick Button 10"=w109:bool, "Joystick Button 11"=w111:bool, "Joystick Button 12"=w110:bool)  [unwired: 1 out]
        n84 = global write "Robot Global Data.vi" "Auto Butt 1"(w116) -> ()
        n85 = global write "Robot Global Data.vi" "Auto Butt 3"(w115) -> ()
        n86 = global write "Robot Global Data.vi" "Auto Butt 5"(w114) -> ()
        n87 = global write "Robot Global Data.vi" "Auto Butt 7"(w113) -> ()
        n88 = global write "Robot Global Data.vi" "Auto Butt 9"(w112) -> ()
        n89 = global write "Robot Global Data.vi" "Auto Butt 11"(w111) -> ()
        n90 = call-poly <vilib>:"WPI_RobotDriveArcadeDrive.vi"("Y axis value"=w120, "X axis value"=w121, "RobotDriveDevRef"=w119) -> ("Motor Values"=w123:dbl[], "RobotDriveDevRef"=w122:T7)  [unwired: 1 in, 6 out]
        n91 = call <vilib>:"WPI_RobotDriveDelayAndUpdateSafety.vi"("Delay (s)"=w117, "RobotDriveDevRef"=w122) -> ("RobotDriveDevRef 2"=w118:T7)  [unwired: 8 in, 1 out]
        n92 = global write "Robot Global Data.vi" "Auto Butt 2"(w105) -> ()
        n93 = global write "Robot Global Data.vi" "Auto Butt 4"(w106) -> ()
        n94 = global write "Robot Global Data.vi" "Auto Butt 6"(w107) -> ()
        n95 = global write "Robot Global Data.vi" "Auto Butt 8"(w108) -> ()
        n96 = global write "Robot Global Data.vi" "Auto Butt 10"(w109) -> ()
        n97 = global write "Robot Global Data.vi" "Auto Butt 12"(w110) -> ()
        n98 = call-poly <vilib>:"SD Write Value.vi"("Numeric Array"=w123) -> ()  [unwired: 9 in, 2 out]
      }
    }
  }
  n99 = case shown="True" w9 {
    frame False {
    }
    frame True {
      # "3"
      n100 = call <vilib>:"WPI_RobotDriveRefNum Registry Get.vi"("refnum name"="Left and Right Motors") -> ("RobotDriveDevRef"=w125:T7)  [unwired: 1 in, 9 out]
      n101 = for {
        tunnel: "Array of robot movements 3" -> [w147] mode=indexing
        tunnel: [w147] -> _ mode=indexing
        tunnel: w125 -> [w144]
        tunnel: [w141] -> _ mode=indexing
        n102 = Unbundle By Name(w147) -> ("X Joystick Value"=w143:dbl, "Y Joystick Value"=w142:dbl, "Delay (sec)"=w140:dbl, "Joystick Button 1"=w139:bool, "Joystick Button 2"=w128:bool, "Joystick Button 3"=w129:bool, "Joystick Button 4"=w130:bool, "Joystick Button 5"=w131:bool, "Joystick Button 6"=w132:bool, "Joystick Button 7"=w133:bool, "Joystick Button 8"=w134:bool, "Joystick Button 9"=w135:bool, "Joystick Button 10"=w136:bool, "Joystick Button 11"=w137:bool, "Joystick Button 12"=w138:bool)  [unwired: 1 out]
        n103 = global write "Robot Global Data.vi" "Auto Butt 1"(w139) -> ()
        n104 = global write "Robot Global Data.vi" "Auto Butt 3"(w129) -> ()
        n105 = global write "Robot Global Data.vi" "Auto Butt 5"(w131) -> ()
        n106 = global write "Robot Global Data.vi" "Auto Butt 7"(w133) -> ()
        n107 = global write "Robot Global Data.vi" "Auto Butt 9"(w135) -> ()
        n108 = global write "Robot Global Data.vi" "Auto Butt 11"(w137) -> ()
        n109 = call-poly <vilib>:"WPI_RobotDriveArcadeDrive.vi"("Y axis value"=w142, "X axis value"=w143, "RobotDriveDevRef"=w144) -> ("Motor Values"=w146:dbl[], "RobotDriveDevRef"=w145:T7)  [unwired: 1 in, 6 out]
        n110 = call <vilib>:"WPI_RobotDriveDelayAndUpdateSafety.vi"("Delay (s)"=w140, "RobotDriveDevRef"=w145) -> ("RobotDriveDevRef 2"=w141:T7)  [unwired: 8 in, 1 out]
        n111 = global write "Robot Global Data.vi" "Auto Butt 2"(w128) -> ()
        n112 = global write "Robot Global Data.vi" "Auto Butt 4"(w130) -> ()
        n113 = global write "Robot Global Data.vi" "Auto Butt 6"(w132) -> ()
        n114 = global write "Robot Global Data.vi" "Auto Butt 8"(w134) -> ()
        n115 = global write "Robot Global Data.vi" "Auto Butt 10"(w136) -> ()
        n116 = global write "Robot Global Data.vi" "Auto Butt 12"(w138) -> ()
        n117 = call-poly <vilib>:"SD Write Value.vi"("Numeric Array"=w146) -> ()  [unwired: 9 in, 2 out]
      }
    }
  }
  n118 = case shown="True" w7 {
    frame False {
    }
    frame True {
      # "4"
      n119 = call <vilib>:"WPI_RobotDriveRefNum Registry Get.vi"("refnum name"="Left and Right Motors") -> ("RobotDriveDevRef"=w148:T7)  [unwired: 1 in, 9 out]
      n120 = for {
        tunnel: "Array of robot movements 4" -> [w170] mode=indexing
        tunnel: [w170] -> _ mode=indexing
        tunnel: w148 -> [w167]
        tunnel: [w164] -> _ mode=indexing
        n121 = Unbundle By Name(w170) -> ("X Joystick Value"=w166:dbl, "Y Joystick Value"=w165:dbl, "Delay (sec)"=w163:dbl, "Joystick Button 1"=w162:bool, "Joystick Button 2"=w156:bool, "Joystick Button 3"=w161:bool, "Joystick Button 4"=w155:bool, "Joystick Button 5"=w160:bool, "Joystick Button 6"=w154:bool, "Joystick Button 7"=w159:bool, "Joystick Button 8"=w153:bool, "Joystick Button 9"=w158:bool, "Joystick Button 10"=w152:bool, "Joystick Button 11"=w157:bool, "Joystick Button 12"=w151:bool)  [unwired: 1 out]
        n122 = global write "Robot Global Data.vi" "Auto Butt 1"(w162) -> ()
        n123 = global write "Robot Global Data.vi" "Auto Butt 3"(w161) -> ()
        n124 = global write "Robot Global Data.vi" "Auto Butt 5"(w160) -> ()
        n125 = global write "Robot Global Data.vi" "Auto Butt 7"(w159) -> ()
        n126 = global write "Robot Global Data.vi" "Auto Butt 9"(w158) -> ()
        n127 = global write "Robot Global Data.vi" "Auto Butt 11"(w157) -> ()
        n128 = call-poly <vilib>:"WPI_RobotDriveArcadeDrive.vi"("Y axis value"=w165, "X axis value"=w166, "RobotDriveDevRef"=w167) -> ("Motor Values"=w169:dbl[], "RobotDriveDevRef"=w168:T7)  [unwired: 1 in, 6 out]
        n129 = call <vilib>:"WPI_RobotDriveDelayAndUpdateSafety.vi"("Delay (s)"=w163, "RobotDriveDevRef"=w168) -> ("RobotDriveDevRef 2"=w164:T7)  [unwired: 8 in, 1 out]
        n130 = global write "Robot Global Data.vi" "Auto Butt 2"(w156) -> ()
        n131 = global write "Robot Global Data.vi" "Auto Butt 4"(w155) -> ()
        n132 = global write "Robot Global Data.vi" "Auto Butt 6"(w154) -> ()
        n133 = global write "Robot Global Data.vi" "Auto Butt 8"(w153) -> ()
        n134 = global write "Robot Global Data.vi" "Auto Butt 10"(w152) -> ()
        n135 = global write "Robot Global Data.vi" "Auto Butt 12"(w151) -> ()
        n136 = call-poly <vilib>:"SD Write Value.vi"("Numeric Array"=w169) -> ()  [unwired: 9 in, 2 out]
      }
    }
  }
  n137 = case shown="True" w3 {
    frame False {
    }
    frame True {
      n138 = call <vilib>:"WPI_RobotDriveRefNum Registry Get.vi"("refnum name"="Left and Right Motors") -> ("RobotDriveDevRef"=w172:T7)  [unwired: 1 in, 9 out]
      n139 = for {
        tunnel: [w193] -> _ mode=indexing
        tunnel: "Array of robot movements 1" -> [w193] mode=indexing
        tunnel: w172 -> [w192]
        tunnel: [w187] -> _ mode=indexing
        n140 = Unbundle By Name(w193) -> ("X Joystick Value"=w191:dbl, "Y Joystick Value"=w190:dbl, "Delay (sec)"=w186:dbl, "Joystick Button 1"=w179:bool, "Joystick Button 2"=w178:bool, "Joystick Button 3"=w177:bool, "Joystick Button 4"=w180:bool, "Joystick Button 5"=w176:bool, "Joystick Button 6"=w181:bool, "Joystick Button 7"=w175:bool, "Joystick Button 8"=w182:bool, "Joystick Button 9"=w174:bool, "Joystick Button 10"=w183:bool, "Joystick Button 11"=w184:bool, "Joystick Button 12"=w185:bool)  [unwired: 1 out]
        n141 = global write "Robot Global Data.vi" "Auto Butt 1"(w179) -> ()
        n142 = global write "Robot Global Data.vi" "Auto Butt 3"(w177) -> ()
        n143 = global write "Robot Global Data.vi" "Auto Butt 5"(w176) -> ()
        n144 = global write "Robot Global Data.vi" "Auto Butt 7"(w175) -> ()
        n145 = global write "Robot Global Data.vi" "Auto Butt 9"(w174) -> ()
        n146 = global write "Robot Global Data.vi" "Auto Butt 11"(w184) -> ()
        n147 = call-poly <vilib>:"WPI_RobotDriveArcadeDrive.vi"("Y axis value"=w190, "X axis value"=w191, "RobotDriveDevRef"=w192) -> ("Motor Values"=w189:dbl[], "RobotDriveDevRef"=w188:T7)  [unwired: 1 in, 6 out]
        n148 = global write "Robot Global Data.vi" "Auto Butt 2"(w178) -> ()
        n149 = global write "Robot Global Data.vi" "Auto Butt 4"(w180) -> ()
        n150 = global write "Robot Global Data.vi" "Auto Butt 6"(w181) -> ()
        n151 = global write "Robot Global Data.vi" "Auto Butt 8"(w182) -> ()
        n152 = global write "Robot Global Data.vi" "Auto Butt 10"(w183) -> ()
        n153 = global write "Robot Global Data.vi" "Auto Butt 12"(w185) -> ()
        n154 = call <vilib>:"WPI_RobotDriveDelayAndUpdateSafety.vi"("Delay (s)"=w186, "RobotDriveDevRef"=w188) -> ("RobotDriveDevRef 2"=w187:T7)  [unwired: 8 in, 1 out]
        n155 = call-poly <vilib>:"SD Write Value.vi"("Numeric Array"=w189) -> ()  [unwired: 9 in, 2 out]
      }
    }
  }
